vi "Averager Compute.vi"(8 "error in (no error)":errorcluster, 10 "Data":dbl[](array[numeric]), 11 "Standard Averager in":refnum<class "Standard Averager.lvclass">) -> (0 "error out":errorcluster, 3 "Standard Averager out":refnum<class "Standard Averager.lvclass">)   [LabVIEW 2018, in "Standard Averager.lvclass"]
uses:
  Standard Averager.lvclass
  C:/Users/aaron.jencks/Documents/GitHub/emerson_seed_object_detection/LabVIEW/Projects/Paul's Video Viewer/Classes/Averager/Averager.lvclass
  <vilib>/Analysis/NI_AALBase.lvlib
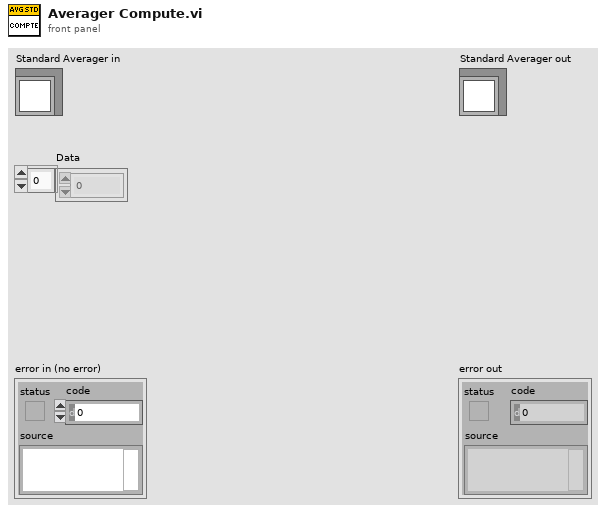
[diagram p1: front panel]
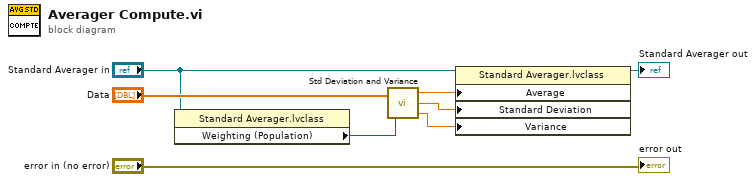
[diagram p0: block diagram]
diagram:
  n1 = property class="Standard Averager.lvclass"(reference="Standard Averager in") -> ("Weighting (Population)"=w1:enum16{"Sample", "Population"})  [unwired: 1 in, 2 out]
  n2 = call <vilib>:"Std Deviation and Variance.vi"("X"="Data", "Weighting (Sample)"=w1) -> ("mean"=w6:dbl, "standard deviation"=w4:dbl, "variance"=w3:dbl)
  n3 = property class="Standard Averager.lvclass"(reference="Standard Averager in", "Average"=w6, "Standard Deviation"=w4, "Variance"=w3) -> (reference out=→"Standard Averager out":refnum<class "Standard Averager.lvclass">)  [unwired: 1 in, 1 out]
  "error out" <- "error in (no error)"
